vi "Loop wait test.vi"() -> ()   [LabVIEW 2020]
uses:
  PPL/HDH.Actor Framework.Core.Sequencer.lvlibp/Sequencer/Sequencer.lvclass
  C:/Current projects/WS/PPL/HDH.Actor Framework.Core.Actor.lvlibp/1abvi3w/vi.lib/ActorFramework/Actor/Actor.lvclass
  PPL/HDH.Actor Framework.Core.Msg.lvlibp/Show Actor Msg/Show Actor Msg.lvclass
  C:/Current projects/WS/PPL/HDH.Actor Framework.Core.Actor.lvlibp/1abvi3w/vi.lib/ActorFramework/Message/Message.lvclass
  PPL/HDH.Actor Framework.Core.Sequencer.lvlibp/Sequencer Messages/Batch Msg/Batch Msg.lvclass
  PPL/HDH.Actor Framework.Core.Sequencer.lvlibp
  PPL/HDH.Actor Framework.Core.Actor.lvlibp/1abvi3w/vi.lib/ActorFramework/Actor/Actor.lvclass
  PPL/HDH.Actor Framework.Core.Actor.lvlibp/1abvi3w/vi.lib/ActorFramework/Message Enqueuer/Message Enqueuer.lvclass
  PPL/HDH.Actor Framework.Core.Actor.lvlibp/1abvi3w/vi.lib/ActorFramework/Stop Msg/Stop Msg.lvclass
  PPL/HDH.Actor Framework.Core.Sequencer.lvlibp/Sequencer Messages/Wait Msg/Wait Msg.lvclass
  PPL/HDH.Actor Framework.Core.Sequencer.lvlibp/Sequencer Messages/Loop Msg/Loop Msg.lvclass
  PPL/HDH.Actor Framework.Core.Sequencer.lvlibp/Sequence Editor/Controls/Ctl_FlexDataElement.ctl
  PPL/HDH.Actor Framework.Core.Sequencer.lvlibp/Sequence Editor/Controls/Ctl_FlexDataElements.ctl
  C:/Current projects/WS/PPL/HDH.Actor Framework.Core.Sequencer.lvlibp/Sequencer Messages/Batch Msg/Batch Msg.lvclass
panel:
  in  "Tree":string(tree)
  in  "Stop Sequencer":bool
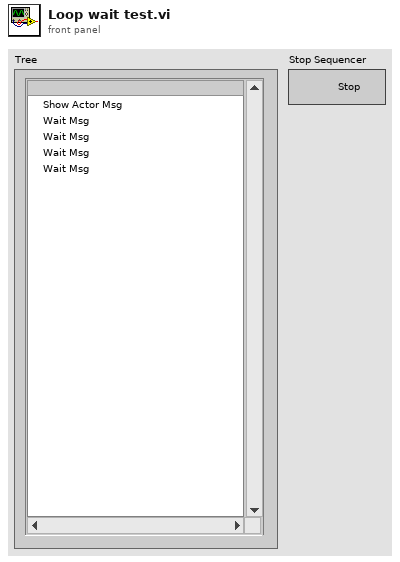
[diagram p1: front panel]
types:
  T1 = typedef "HDH.Actor Framework.Core.Sequencer.lvlibp/Ctl_FlexDataElement.ctl" = cluster{"Control Index":i32, "Data Values":variant[]}
  T2 = typedef "HDH.Actor Framework.Core.Sequencer.lvlibp/Ctl_FlexDataElements.ctl" = cluster{"Flex Data":T1[]}
  T3 = typedef "HDH.Actor Framework.Core.Sequencer.lvlibp/Ctl_SequenceElement.ctl" = cluster{"Message Base Name":string, "Message Path":path, "Supports Data Access?":bool, "List Symbol":i32, "Sequence Control Element Array":T4[]}
  T4 = typedef "HDH.Actor Framework.Core.Sequencer.lvlibp/Ctl_SequenceControlElement.ctl" = cluster{"Data Override name":string, "Looped Override?":bool, "Control element":T5, "List Symbol":i32}
  T5 = typedef "HDH.Actor Framework.Core.Msg.lvlibp/Ctl_Control Element.ctl" = cluster{"Index":i32, "Label":string, "Value":variant}
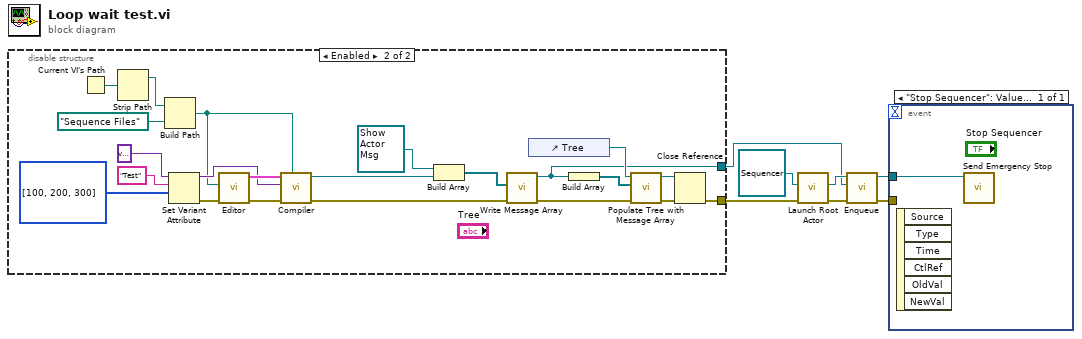
[diagram p0: block diagram]
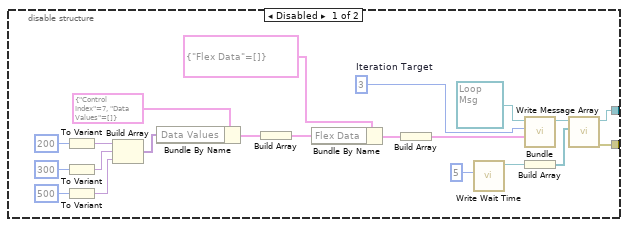
[diagram p2: hidden frame]
diagram:
  n1 = disable-structure shown="Enabled" {
    disable-tunnel: [w9 w35] -> w5
    disable-tunnel: [w8 w40] -> w2
    frame Disabled {
      w27 = 3  # Iteration Target
      n2 = To Variant(anything=200 ("Iteration Target")) -> (Variant=w20:variant)
      n3 = To Variant(anything=300 ("Iteration Target")) -> (Variant=w19:variant)
      n4 = To Variant(anything=500 ("Iteration Target")) -> (Variant=w18:variant)
      n5 = Build Array(w20, w19, w18) -> (w16:variant[])
      n6 = Bundle By Name(cluster=T1 {"Control Index"=7, "Data Values"=[]} ("Flex Data Element"), "Data Values"=w16) -> (w17:T1)
      n7 = Build Array(w17) -> (w14:T1[])
      n8 = Bundle By Name(cluster=T2 {"Flex Data"=[]} ("Flex Data Elements Cluster Array"), "Flex Data"=w14) -> (w15:T2)
      n9 = Build Array(w15) -> (w25:T2[])
      n10 = call "Write Wait Time.vi"("Wait Time in ms (0)"=5) -> ("Wait Msg out"=w11:refnum<class "Wait Msg.lvclass">)  [unwired: 9 in, 1 out]
      n11 = call "Bundle.vi"("Override data"=w25, "Iteration Target"=w27, "Loop Msg in"=refnum<class "Loop Msg.lvclass"> refnum ("HDH.Actor Framework.Core.Sequencer.lvlibp:Loop Msg.lvclass")) -> ("Loop Msg out"=w13:refnum<class "Loop Msg.lvclass">)  [unwired: 7 in, 1 out]
      n12 = Build Array(w11) -> (w10:refnum<class "Wait Msg.lvclass">[])
      n13 = call "Write Message Array.vi"("Message Array"=w10, "Batch Msg in"=w13) -> ("error out"=w8:errorcluster, "Batch Msg out"=w9:refnum<class "Loop Msg.lvclass">)  [unwired: 8 in]
    }
    frame Enabled {
      n14 = Current VI's Path() -> (path=w32:path)
      n15 = Strip Path(path=w32) -> (stripped path=w31:path)  [unwired: 1 out]
      n16 = Build Path(base path=w31, name or relative path=path "Sequence Files" ("Sequence folder path")) -> (appended path=w29:path)
      n17 = Set Variant Attribute(Variant=variant, name="Test", value=i32[] [100, 200, 300]) -> (Variant out=w45:variant, error out=w44:errorcluster)  [unwired: 1 in, 1 out]
      n18 = call "Editor.vi"("error in (no error)"=w44, "Browse start path"=w29) -> ("error out"=w49:errorcluster, "Uncompiled sequence out"=w50:T3[])  [unwired: 8 in]
      n19 = call "Compiler.vi"("Sequence folder path"=w29, "error in (no error)"=w49, "Override Look up table"=w45, "Uncompiled sequence in"=w50) -> ("error out"=w34:errorcluster, "Batch Msg out"=w43:refnum<class "Batch Msg.lvclass">)  [unwired: 5 in, 1 out]
      n20 = Build Array(refnum<class "Show Actor Msg.lvclass"> refnum ("HDH.Actor Framework.Core.Msg.lvlibp:Show Actor Msg.lvclass"), w43) -> (w37:refnum<class "Message.lvclass">[])
      n21 = call "Write Message Array.vi"("error in (no error)"=w34, "Message Array"=w37) -> ("error out"=w33:errorcluster, "Batch Msg out"=w35:refnum<class "Batch Msg.lvclass">)  [unwired: 8 in]
      n22 = control-ref of="Tree"() -> (w41:refnum<vi>)
      n23 = Build Array(w35) -> (w36:refnum<class "Batch Msg.lvclass">[])
      n24 = call "Populate Tree with Message Array.vi"("error in (no error)"=w33, "Message Array"=w36, "Tree in"=w41) -> ("error out"=w42:errorcluster, "Tree out"=w39:refnum<vi>)  [unwired: 7 in]
      n25 = Close Reference(reference=w39, error in (no error)=w42) -> (error out=w40:errorcluster)
    }
  }
  n26 = call "Launch Root Actor.vi"("error in (no error)"=w2, "Actor"=refnum<class "Sequencer.lvclass"> refnum ("HDH.Actor Framework.Core.Sequencer.lvlibp:Sequencer.lvclass")) -> ("error out"=w1:errorcluster, "Actor's Enqueuer"=w6:refnum<class "Message Enqueuer.lvclass">)  [unwired: 8 in]
  n27 = call "Enqueue.vi"("error in (no error)"=w1, "Message"=w5, "Message Enqueuer in"=w6) -> ("error out"=w4:errorcluster, "Message Enqueuer out"=w3:refnum<class "Message Enqueuer.lvclass">)  [unwired: 7 in]
  n28 = event shown="[0] \"Stop Sequencer\": Value Change" {
    selector: _ -> [_]
    dyn-events: _ -> [_]
    timeout: _ -> [_]
    tunnel: w4 -> [_]
    tunnel: w3 -> [w51]
    event "Stop Sequencer": Value Change {
      n29 = event-data() -> ()  [unwired: 1 in, 6 out]
      n30 = call "Send Emergency Stop.vi"("Message Enqueuer"=w51) -> ()  [unwired: 10 in, 1 out]
    }
  }
